vi "Memory.Pointer.Swap.Safe.vi"(8 "error in (no error)":errorcluster, 10 "pointer b":refnum<class "Memory.Pointer.lvclass">, 11 "pointer a":refnum<class "Memory.Pointer.lvclass">) -> (0 "error out":errorcluster, 2 "pointer b":refnum<class "Memory.Pointer.lvclass">, 3 "pointer a":refnum<class "Memory.Pointer.lvclass">)   [LabVIEW 2016, in "Memory Manager.lvlib" / "Memory.Pointer.lvclass"]
uses:
  Memory.Pointer.lvclass
  Memory.Pointer.lvclass/Memory.Pointer.ctl
  Accessors/Get Address.vi
  Accessors/Set Address.vi
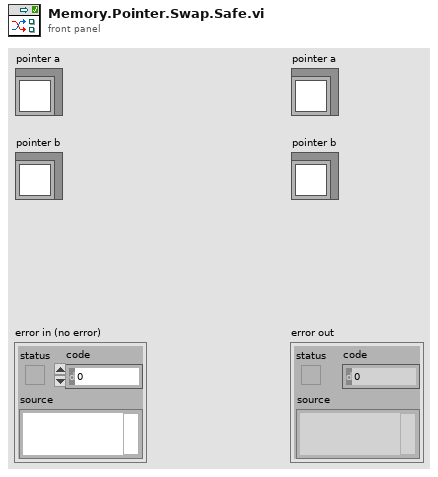
[diagram p1: front panel]
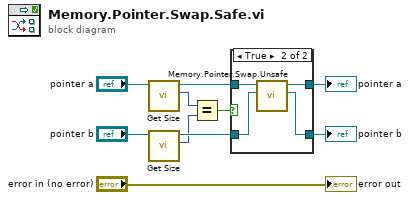
[diagram p0: block diagram]
diagram:
  n1 = call "Get Size.vi"("Pointer in"="pointer a") -> ("size"=w7:u64, "Pointer out"=w5:refnum<class "Memory.Pointer.lvclass">)  [unwired: 8 in, 1 out]
  n2 = call "Get Size.vi"("Pointer in"="pointer b") -> ("size"=w3:u64, "Pointer out"=w4:refnum<class "Memory.Pointer.lvclass">)  [unwired: 8 in, 1 out]
  n3 = Equal?(x=w7, y=w3) -> (x = y?=w6:bool)
  n4 = case shown="True" w6 {
    tunnel: w5 -> [w12 w16]
    tunnel: w4 -> [w11 w14]
    tunnel: [w12 w15] -> w2
    tunnel: [w11 w13] -> w1
    frame False {
    }
    frame True {
      n5 = call "Memory.Pointer.Swap.Unsafe.vi"("pointer b"=w14, "pointer a"=w16) -> ("pointer b"=w13:refnum<class "Memory.Pointer.lvclass">, "pointer a"=w15:refnum<class "Memory.Pointer.lvclass">)  [unwired: 7 in, 1 out]
    }
  }
  "pointer a" <- w2
  "pointer b" <- w1
  "error out" <- "error in (no error)"
